vi "Focus Point.vi"(4 "Zoom Factor":dbl, 6 "Transformation Matrix":T1, 8 "error in":errorcluster, 9 "FOV":cluster{"X [um]":dbl, "Y [um]":dbl} {"Y [um]" format="%.2f"; "X [um]" format="%.2f"}, 10 "Target Coordinates":T2, 11 "GFG Refnum":refnum<vi>) -> (0 "error out":errorcluster, 3 "GFG Refnum Out":refnum<vi>)   [LabVIEW 2012, in "Sciscan Scope Daemon.lvlib"]
uses:
  Sciscan Scope Daemon.lvlib
  <vilib>/Analysis/Matrix/Datatypes/RealMatrix.ctl
  <vilib>/Analysis/Matrix/Numeric/Absolute Value/Absolute Value - RM.vi
  <vilib>/Analysis/Matrix/Numeric/Add/Add - RM,RM.vi
  <vilib>/Analysis/baseanly.llb/Real A x B.vi
  <vilib>/Analysis/NI_AALBase.lvlib
  <vilib>/Analysis/Matrix/NI_Matrix.lvlib
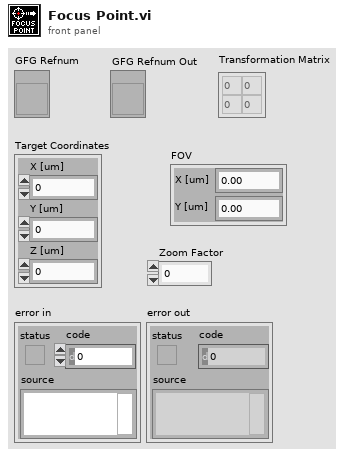
[diagram p1: front panel]
types:
  T1 = typedef "NI_Matrix.lvlib/RealMatrix.ctl" = dbl[][]
  T2 = cluster{"X [um]":dbl, "Y [um]":dbl, "Z [um]":dbl}
  T3 = cluster{"X [um]":bool, "Y [um]":bool, "Z [um]":bool}
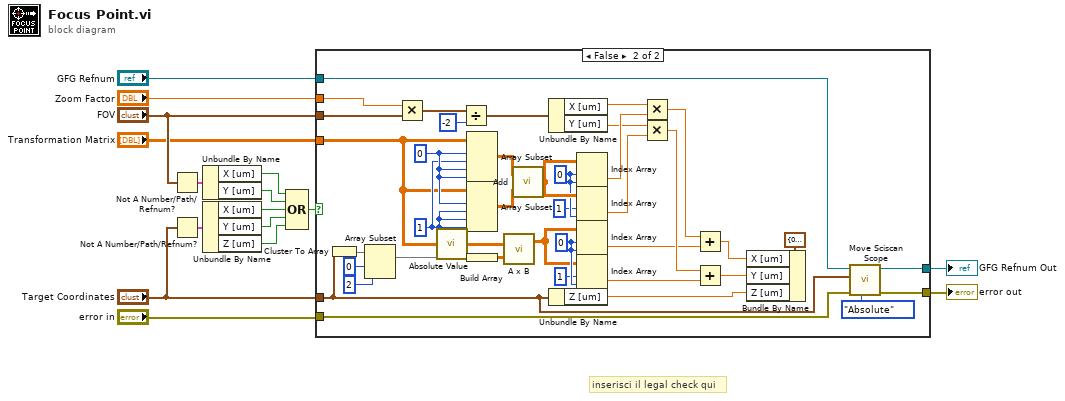
[diagram p0: block diagram]
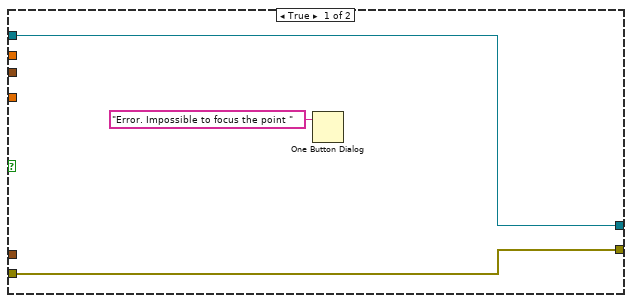
[diagram p2: hidden frame]
diagram:
  # "inserisci il legal check qui"
  n1 = Not A Number/Path/Refnum?(number/path/refnum="FOV") -> (NaN/Path/Refnum?=w14:cluster{"X [um]":bool, "Y [um]":bool})
  n2 = Not A Number/Path/Refnum?(number/path/refnum="Target Coordinates") -> (NaN/Path/Refnum?=w15:T3)
  n3 = Unbundle By Name(w14) -> ("X [um]"=w12:bool, "Y [um]"=w11:bool)
  n4 = Unbundle By Name(w15) -> ("X [um]"=w10:bool, "Y [um]"=w9:bool, "Z [um]"=w8:bool)
  n5 = Compound Arithmetic op=OR(w12, w11, w10, w9, w8) -> (w6:bool)
  n6 = case shown="False" w6 {
    tunnel: [w19 w58] -> w4
    tunnel: [w18 w57] -> w16
    tunnel: "Target Coordinates" -> [_ w20]
    tunnel: "FOV" -> [_ w23]
    tunnel: "GFG Refnum" -> [w19 w59]
    tunnel: "error in" -> [w18 w56]
    tunnel: "Transformation Matrix" -> [_ w30]
    tunnel: "Zoom Factor" -> [_ w28]
    frame True {
      n7 = One Button Dialog(message="Error. Impossible to focus the point " ("Window Title (\"\")")) -> ()  [unwired: 1 in, 1 out]
    }
    frame False {
      w35 = 0 ("index (row)")
      w41 = 0 ("index (row)")
      w44 = 1 ("row N")
      w45 = 0 ("row 1")
      n8 = Cluster To Array(cluster=w20) -> (array=w52:dbl[])
      n9 = Array Subset(array=w52, index=0, length=2) -> (w51:dbl[])
      n10 = Multiply(x=w28, y=w23) -> (x*y=w22:cluster{"X [um]":dbl, "Y [um]":dbl})
      n11 = call-poly <vilib>:"Absolute Value.vi"("Real Matrix A"=w30) -> ("|A|"=w29:T1)
      n12 = Divide(x=w22, y=-2) -> (x/y=w21:cluster{"X [um]":dbl, "Y [um]":dbl})
      n13 = Array Subset(array=w30, index (row)=w45, length (row)=w44, index (col)=w45, length (col)=w45) -> (w47:T1)
      n14 = Array Subset(array=w30, index (row)=w45, length (row)=w44, index (col)=w44, length (col)=w44) -> (w46:T1)
      n15 = Build Array(w51) -> (w48:T1)
      n16 = call-poly <vilib>:"A x B.vi"("B"=w48, "A"=w29) -> ("A x B"=w33:T1)  [unwired: 1 out]
      n17 = call-poly <vilib>:"Add.vi"("Real Matrix B"=w46, "Real Matrix A"=w47) -> ("A + B"=w42:T1)
      n18 = Unbundle By Name(w21) -> ("X [um]"=w39:dbl, "Y [um]"=w37:dbl)
      n19 = Unbundle By Name(w20) -> ("Z [um]"=w53:dbl)
      n20 = Index Array(array=w42, index (row)=w41, index (col)=w41) -> (element=w38:dbl)
      n21 = Index Array(array=w42, index (row)=1 ("index (col)"), index (col)=w41) -> (element=w36:dbl)
      n22 = Index Array(array=w33, index (row)=w35, index (col)=w35) -> (element=w27:dbl)
      n23 = Index Array(array=w33, index (row)=1 ("index (col)"), index (col)=w35) -> (element=w26:dbl)
      n24 = Multiply(x=w39, y=w38) -> (x*y=w32:dbl)
      n25 = Multiply(x=w37, y=w36) -> (x*y=w31:dbl)
      n26 = Add ("Add.vi")(x=w32, y=w27) -> (x+y=w25:dbl)
      n27 = Add ("Add.vi")(x=w31, y=w26) -> (x+y=w24:dbl)
      n28 = Bundle By Name(cluster=T2 {"X [um]"=0.0, "Y [um]"=0.0, "Z [um]"=0.0} ("x/y"), "X [um]"=w25, "Y [um]"=w24, "Z [um]"=w53) -> ()  [unwired: 1 out]
      n29 = call "Move Sciscan Scope.vi"("Type"=enum16{"Relative", "Absolute"}."Absolute", "error in"=w56, "Displacement [um]"=w20, "GFG Refnum"=w59) -> ("error out"=w57:errorcluster, "GFG Refnum Out"=w58:refnum<vi>)  [unwired: 6 in]
    }
  }
  "error out" <- w16
  "GFG Refnum Out" <- w4
